vi "BoilerStateMachine.vi"() -> ()   [LabVIEW 2023]
uses:
  <vilib>/Utility/error.llb/Trim Whitespace One-Sided.vi
  Heater.vi
  AC.vi
panel:
  out "Waveform Chart 2":dbl[][](graph)
  out "Waveform Chart":i32(graph)
  out "Message":string
  out "Alarm":bool
  out "Temperature":dbl
  in  "?":dbl(knob) min=0.0 max=2.0 step=1.0 scale=0.0..2.0
  in  "stop":bool
  out "Thermometer":dbl(slide) scale=0.0..100.0
  in  "Min temperature":dbl=20.0
  in  "Max temperature":dbl=80.0
  in  "Automatic / Manual":bool
  out "Cooling":bool
  out "Heater":bool
  # "Heater"
  # "Off"
  # "Cooling"
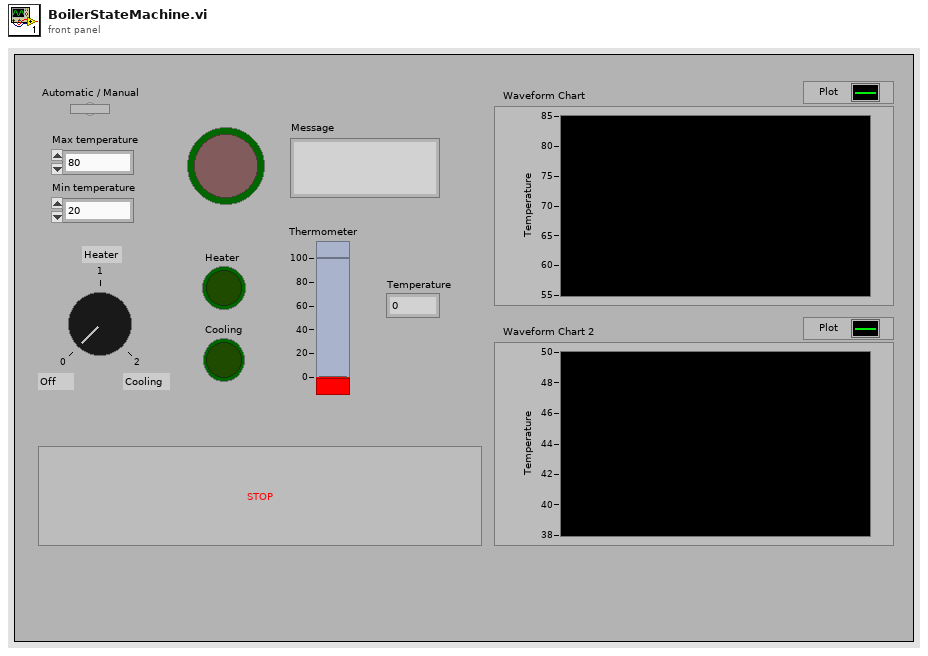
[diagram p1: front panel]
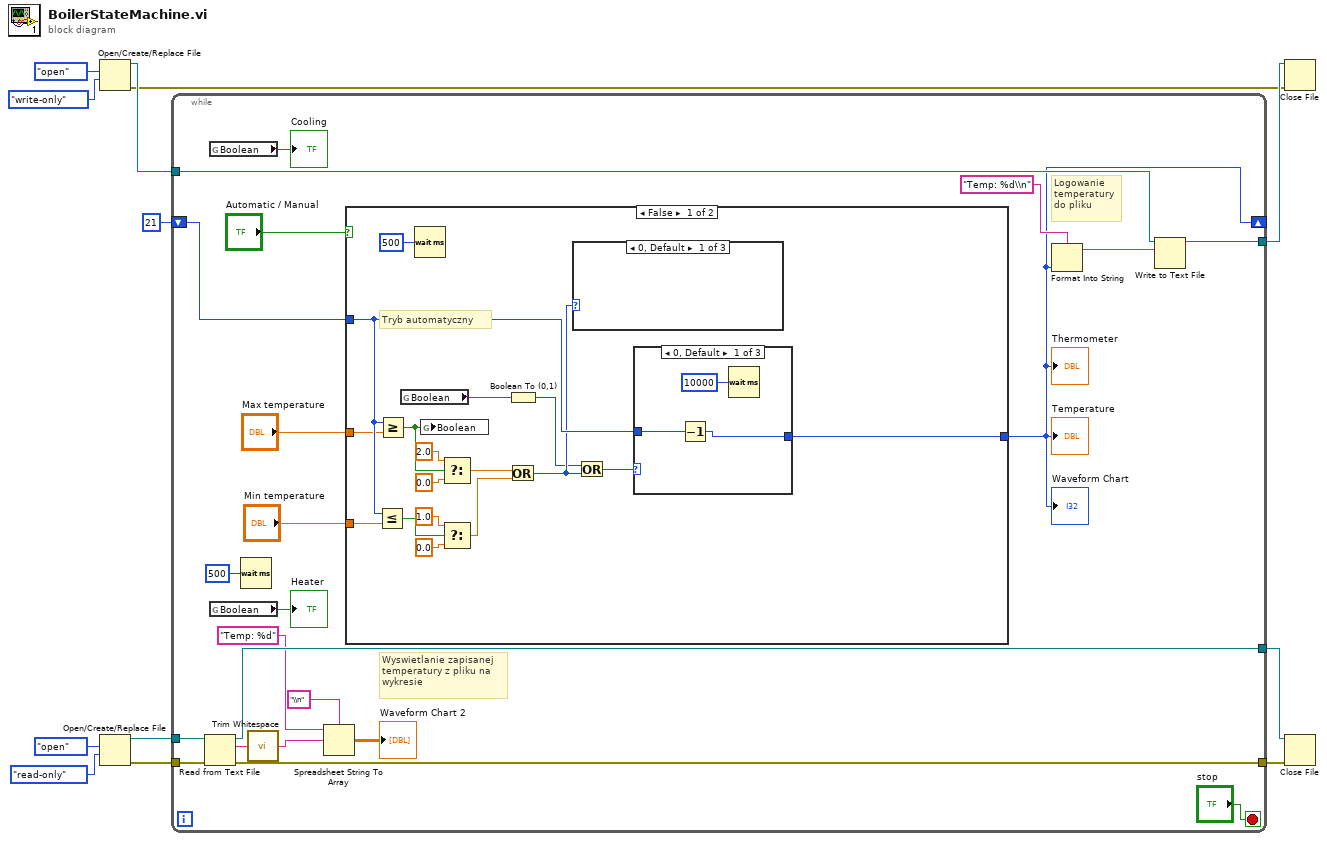
[diagram p0: block diagram]
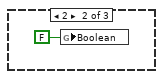
[diagram p2: hidden frame]
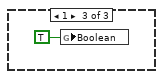
[diagram p3: hidden frame]
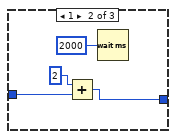
[diagram p4: hidden frame]
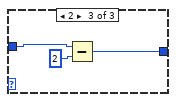
[diagram p5: hidden frame]
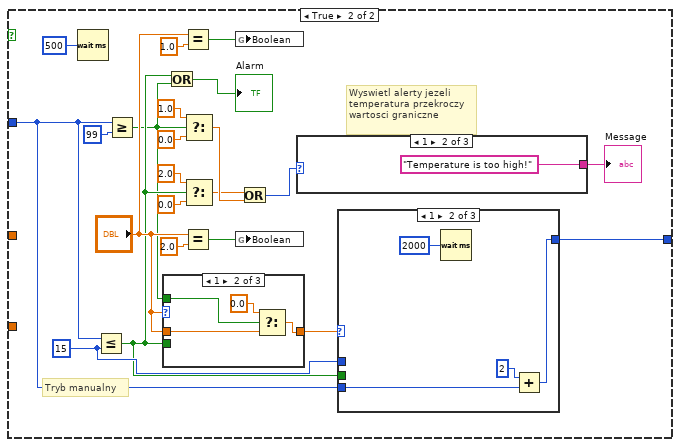
[diagram p6: hidden frame]
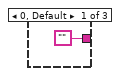
[diagram p7: hidden frame]
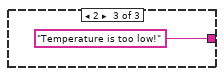
[diagram p8: hidden frame]
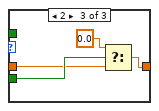
[diagram p10: hidden frame]
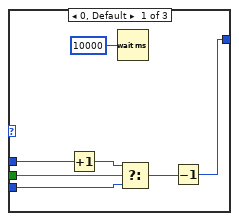
[diagram p11: hidden frame]
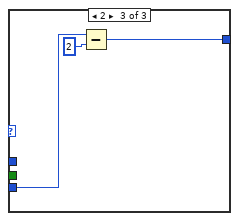
[diagram p12: hidden frame]
diagram:
  n1 = Open/Create/Replace File(operation (0:open)=enum16{"open", "replace"}."open", access (0:read/write)=enum16{"read/write", "read-only", "write-only"}."write-only") -> (refnum out=w8:refnum<file>, error out=w7:errorcluster)  [unwired: 4 in, 1 out]
  n2 = Open/Create/Replace File(operation (0:open)=enum16{"open", "replace"}."open", access (0:read/write)=enum16{"read/write", "read-only", "write-only"}."read-only") -> (refnum out=w3:refnum<file>, error out=w4:errorcluster)  [unwired: 4 in, 1 out]
  n3 = while {
    shift-right: [w23] -> _
    shift-left: 21 -> [w27]
    tunnel: w8 -> [w26]
    tunnel: [w25] -> w10
    tunnel: w4 -> [w21]
    tunnel: w3 -> [w20]
    tunnel: [w19] -> w2
    tunnel: [w18] -> w1
    stop <- "stop" stop-if-true
    # "Wyswietlanie zapisanej temperatury z pliku na wykresie"
    # "Logowanie temperatury do pliku"
    n4 = Read from Text File(file (use dialog)=w20, error in=w21) -> (refnum out=w18:refnum<file>, text=w17:string, error out=w19:errorcluster)  [unwired: 2 in, 1 out]
    n5 = global read "AC.vi" "Boolean"() -> (→"Cooling":bool)
    n6 = global read "Heater.vi" "Boolean"() -> (→"Heater":bool)
    n7 = Wait (ms)(milliseconds to wait=u32 500) -> ()  [unwired: 1 out]
    n8 = call <vilib>:"Trim Whitespace.vi"("string"=w17) -> ("trimmed string"=w13:string)  [unwired: 1 in]
    n9 = Spreadsheet String To Array(delimiter (Tab)="\\n", format string="Temp: %d", spreadsheet string=w13) -> (array=→"Waveform Chart 2":dbl[][])  [unwired: 1 in]
    n10 = case shown="False" "Automatic / Manual" {
      tunnel: w27 -> [w44 w78]
      tunnel: "Max temperature" -> [w43 _]
      tunnel: "Min temperature" -> [w42 _]
      tunnel: [w46 w84] -> w23
      frame False {
        # "Tryb automatyczny"
        n11 = Less Or Equal?(x=w44, y=w42) -> (x <= y?=w39:bool)
        n12 = Greater Or Equal?(x=w44, y=w43) -> (x >= y?=w40:bool)
        n13 = global read "Heater.vi" "Boolean"() -> (w35:bool)
        n14 = Wait (ms)(milliseconds to wait=u32 500) -> ()  [unwired: 1 out]
        n15 = global write "AC.vi" "Boolean"(w40) -> ()
        n16 = Select(t=2.0, s=w40, f=0.0) -> (s? t:f=w47:dbl)
        n17 = Select(t=1.0, s=w39, f=0.0) -> (s? t:f=w41:dbl)
        n18 = Boolean To (0,1)(Boolean=w35) -> (0, 1=w36:i16)
        n19 = Or(x=w47, y=w41) -> (x .or. y?=w38:i32)
        n20 = case shown="0, Default" w38 {
          frame 0, Default {
          }
          frame 2 {
            n21 = global write "Heater.vi" "Boolean"(FALSE ("Boolean")) -> ()
          }
          frame 1 {
            n22 = global write "Heater.vi" "Boolean"(TRUE ("Boolean")) -> ()
          }
        }
        n23 = Or(x=w36, y=w38) -> (x .or. y?=w37:i32)
        n24 = case shown="0, Default" w37 {
          tunnel: w44 -> [w56 w60 w63]
          tunnel: [w55 w58 w62] -> w46
          frame 0, Default {
            n25 = Decrement(x=w56) -> (x-1=w55:i32)
            n26 = Wait (ms)(milliseconds to wait=u32 10000) -> ()  [unwired: 1 out]
          }
          frame 1 {
            n27 = Add(x=2, y=w60) -> (x+y=w58:i32)
            n28 = Wait (ms)(milliseconds to wait=u32 2000) -> ()  [unwired: 1 out]
          }
          frame 2 {
            n29 = Subtract(x=w63, y=2) -> (x-y=w62:i32)
          }
        }
      }
      frame True {
        w75 = 15
        # "Wyswietl alerty jezeli temperatura przekroczy wartosci graniczne"
        # "Tryb manualny"
        n30 = Wait (ms)(milliseconds to wait=u32 500) -> ()  [unwired: 1 out]
        n31 = Less Or Equal?(x=w78, y=w75) -> (x <= y?=w70:bool)
        n32 = Greater Or Equal?(x=w78, y=99 ("x")) -> (x >= y?=w69:bool)
        n33 = case shown="1" "?" {
          tunnel: "?" -> [w89 w90 w95]
          tunnel: [w89 w92 w96] -> w83
          tunnel: w69 -> [_ w93 _]
          tunnel: w70 -> [_ _ w97]
          frame 0, Default {
          }
          frame 1 {
            n34 = Select(t=0.0 ("f"), s=w93, f=w90) -> (s? t:f=w92:dbl)
          }
          frame 2 {
            n35 = Select(t=0.0, s=w97, f=w95) -> (s? t:f=w96:dbl)
          }
        }
        n36 = Or(x=w70, y=w69) -> (x .or. y?=→"Alarm":bool)
        n37 = Equal?(x="?", y=1.0) -> (x = y?=w81:bool)
        n38 = Equal?(x="?", y=2.0) -> (x = y?=w79:bool)
        n39 = Select(t=1.0, s=w69, f=0.0) -> (s? t:f=w66:dbl)
        n40 = Select(t=2.0, s=w70, f=0.0) -> (s? t:f=w65:dbl)
        n41 = global write "Heater.vi" "Boolean"(w81) -> ()
        n42 = global write "AC.vi" "Boolean"(w79) -> ()
        n43 = Or(x=w65, y=w66) -> (x .or. y?=w64:i32)
        n44 = case shown="1" w64 {
          tunnel: ["" "Temperature is too high!" "Temperature is too low!"] -> w68
          frame 0, Default {
          }
          frame 1 {
          }
          frame 2 {
          }
        }
        "Message" <- w68
        n45 = case shown="1" w83 {
          tunnel: w78 -> [w101 w108 w111]
          tunnel: [w104 w107 w110] -> w84
          tunnel: w70 -> [w102 _ _]
          tunnel: w75 -> [w99 _ _]
          frame 0, Default {
            n46 = Increment(x=w99) -> (x+1=w98:i32)
            n47 = Wait (ms)(milliseconds to wait=u32 10000) -> ()  [unwired: 1 out]
            n48 = Select(t=w98, s=w102, f=w101) -> (s? t:f=w100:i32)
            n49 = Decrement(x=w100) -> (x-1=w104:i32)
          }
          frame 1 {
            n50 = Wait (ms)(milliseconds to wait=u32 2000) -> ()  [unwired: 1 out]
            n51 = Add(x=2, y=w108) -> (x+y=w107:i32)
          }
          frame 2 {
            n52 = Subtract(x=w111, y=2) -> (x-y=w110:i32)
          }
        }
      }
    }
    "Thermometer" <- w23
    "Temperature" <- w23
    "Waveform Chart" <- w23
    n53 = Format Into String(format string="Temp: %d\\n", w23) -> (resulting string=w22:string)  [unwired: 2 in, 1 out]
    n54 = Write to Text File(file (use dialog)=w26, text=w22) -> (refnum out=w25:refnum<file>)  [unwired: 2 in, 2 out]
  }
  n55 = Close File(refnum=w10, error in=w7) -> ()  [unwired: 2 out]
  n56 = Close File(refnum=w1, error in=w2) -> ()  [unwired: 2 out]
